vi "Stop.vi"(8 "error in (no error)":errorcluster) -> (0 "error out":errorcluster)   [LabVIEW 2017, in "BOP_VibAPI_6.lvlib"]
uses:
  <vilib>/addons/InsightCM/Devices/Shared/Cms/Fpga/Acquisition/source/subVIs/VibAPI/BOP_VibAPI_6.lvlib
  <vilib>/rvi/eio/common/nirviEmuTemplateMethod_errors.vi
  <vilib>/eio/EIONode/EIONode.xnode
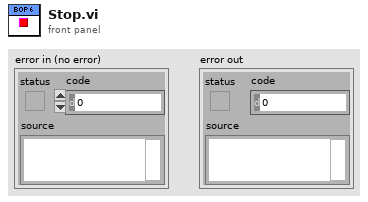
[diagram p1: front panel]
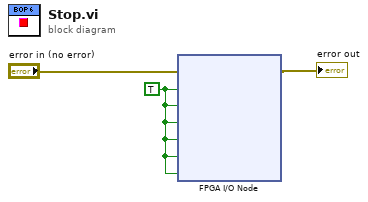
[diagram p0: block diagram]
diagram:
  w3 = TRUE ("Mod1/Stop")
  n1 = xnode "FPGA I/O Node"("error in"="error in (no error)", "Mod1/Stop"=w3, "Mod2/Stop"=w3, "Mod3/Stop"=w3, "Mod4/Stop"=w3, "Mod5/Stop"=w3, "Mod6/Stop"=w3) -> ("error out"=→"error out":errorcluster)  [unwired: 6 in, 6 out]
